vi "Log DAQ Configuration.vi"(8 "error in (no error)":errorcluster, 11 "Instrument.Lockin in":refnum<class "Instrument.Lockin.lvclass">) -> (0 "error out":errorcluster, 3 "Instrument.Lockin out":refnum<class "Instrument.Lockin.lvclass">)   [LabVIEW 2019, in "Instrument.Lockin.lvlib" / "Instrument.Lockin.lvclass"]
uses:
  Instrument.Lockin.lvclass
  C:/Program Files/National Instruments/LabVIEW 2019/user.lib/LevyLab/Instrument Framework/Instrument/Instrument.lvclass
  <userlib>/LevyLab/Instrument Framework/Instrument/Instrument.lvclass
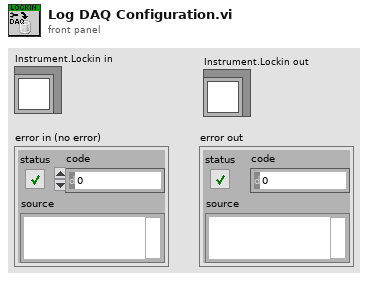
[diagram p1: front panel]
types:
  T1 = typedef "Instrument.Lockin.lvlib/Instrument.Lockin.lvclass/Lockin.LogConfiguration.DAQ--Cluster.ctl" = cluster{"System Serial Number":string, "System Channel":i32, "Chassis Serial Number":string, "Chassis Slot":i32, "Device Serial Number":string, "Device Channel":i32, "Channel Type":string, "Channel Range":string, "Channel Configuration":string, "Temperature":dbl, "Calibration Temperature":dbl, "Calibration Time":string}
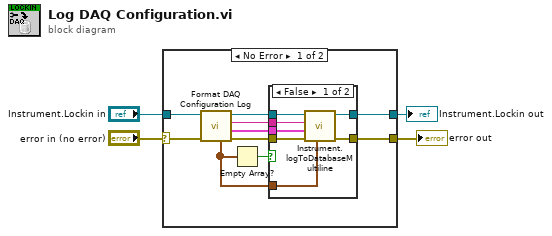
[diagram p0: block diagram]
diagram:
  n1 = case shown="No Error" "error in (no error)" {
    selector: "error in (no error)" -> [w14 w25]
    tunnel: "Instrument.Lockin in" -> [w13 w24]
    tunnel: [w7 w25] -> w3
    tunnel: [w8 w24] -> w1
    frame No Error {
      n2 = call "Format DAQ Configuration Log.vi"("error in (no error)"=w14, "Instrument.Lockin in"=w13) -> ("error out"=w12:errorcluster, "Array"=w11:T1[], "Log Paths"=w10:string, "Instrument.Lockin out"=w9:refnum<class "Instrument.Lockin.lvclass">, "Times"=w5:timestamp[])  [unwired: 5 in]
      n3 = Empty Array?(array=w5) -> (empty?=w6:bool)
      n4 = case shown="False" w6 {
        tunnel: [w21 w23] -> w7
        tunnel: [w20 w22] -> w8
        tunnel: w9 -> [w19 w22]
        tunnel: w10 -> [w18 _]
        tunnel: w11 -> [w17 _]
        tunnel: w5 -> [w16 _]
        tunnel: w12 -> [w15 w23]
        frame False {
          n5 = call <userlib>:"Instrument.logToDatabaseMultiline.vi"("timestamps"=w16, "error in (no error)"=w15, "Data"=w17, "Paths"=w18, "Instrument"=w19) -> ("error out"=w21:errorcluster, "Instrument out"=w20:refnum<class "Instrument.Lockin.lvclass">)  [unwired: 5 in]
        }
        frame True {
        }
      }
    }
    frame Error {
    }
  }
  "error out" <- w3
  "Instrument.Lockin out" <- w1
